vi "Main VI.vi"() -> ()   [LabVIEW 2024]
uses:
  C:/Users/user/Downloads/CarWash-master/CarWash-master/Controls/Wash Options.ctl
  C:/Users/user/Downloads/assignmentFINALHAHA/assignment/TIMEGLOBAL.vi
panel:
  out "Elapsed Time":dbl format="%#.2f"
  out "9. Vehicle Out of Position":bool
  out "8. Air Dry":bool
  out "7. Tire Shine Foam":bool
  out "6. Spot Free Rinse":bool
  out "5. Low Pressure Wax":bool
  out "4. High Pressure Wash":bool
  out "3. Pre-Soak":bool
  out "2. Bug Remover":bool
  out "1. Under Body Wash":bool
  out "Wash Entry":bool
  in  "Start":bool
  in  "Wash Options":T1
  in  "stop program":bool
  in  "Car Position Slider":u8(slide) max=3 scale=0.0..4.0
  # "Car Position Simulation"
  # "Pre-Soak\nH-P Wash\nL-P Wax\nSpot Free Rinse"
  # "Underbody Wash\nBug Remover"
  # "Tire Shine\nAir Dry"
  # "Car Wash Display"
  # "Car Wash Indicators"
  # "Entry Console"
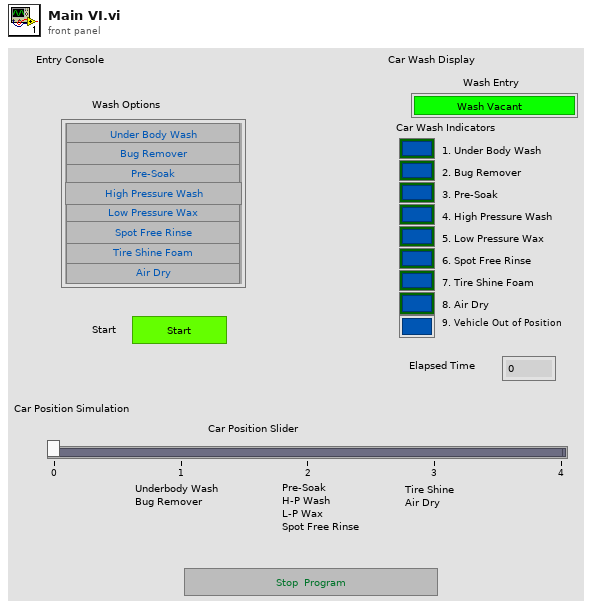
[diagram p1: front panel]
types:
  T1 = typedef "Wash Options.ctl" = cluster{"Underbody Wash":bool, "Bug Remover":bool, "Pre-Soak":bool, "High Pressure Wash":bool, "Low Pressure Wax":bool, "Spot Free Rinse":bool, "Tire Shine Foam":bool, "Air Dry":bool}
  T2 = enum16{"init", "Wait for Start", "Check Position", "under body wash", "bug remover", "pre-soak", "high pressure wash", "low pressure wax", "spot free rinse", "tire shine foam", "air dry", "Check Completion", "Log Data", "Stop Program"}
  T3 = enum8{"Enabled", "Disabled", "Disabled and Grayed Out"}
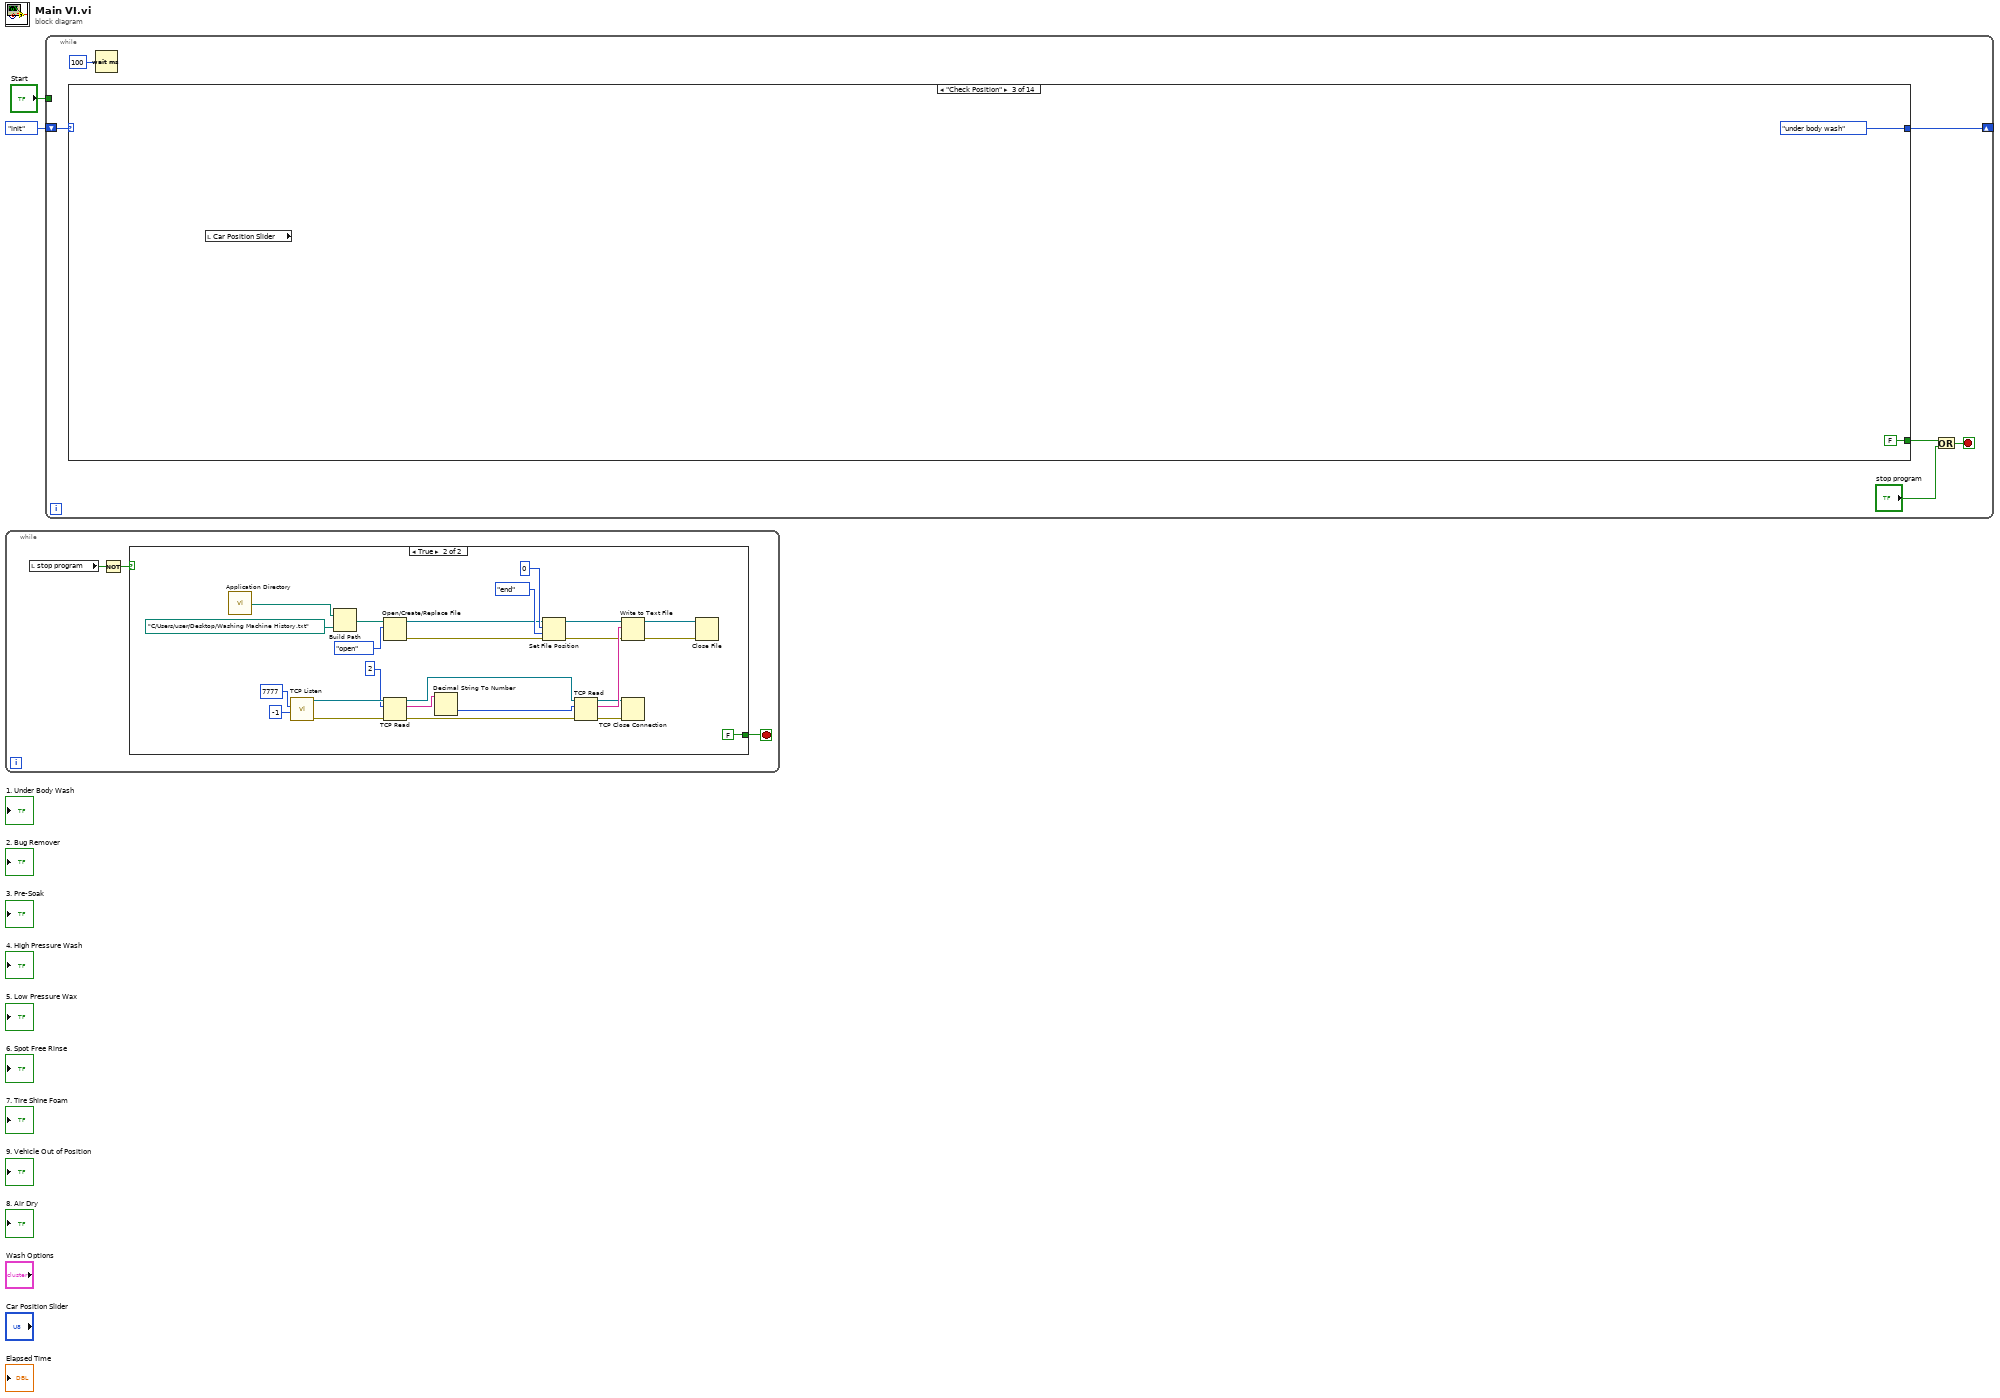
[diagram p0: block diagram]
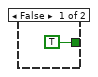
[diagram p2: hidden frame]
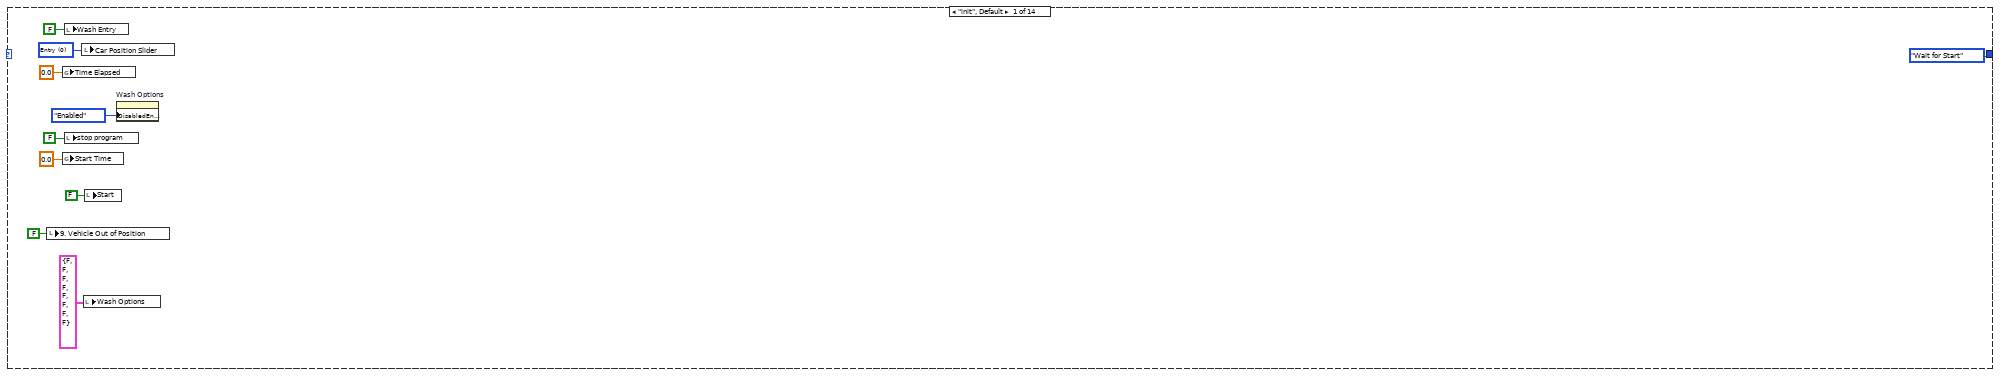
[diagram p3: hidden frame]
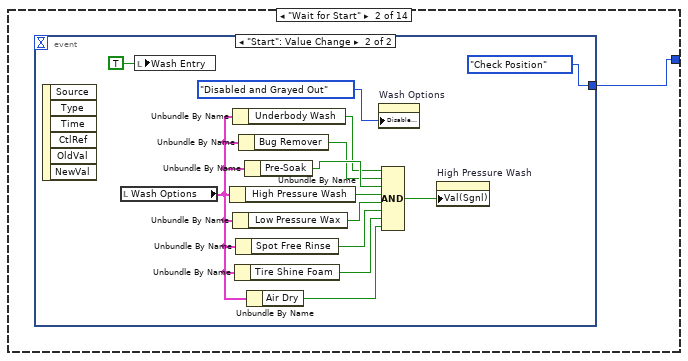
[diagram p4: hidden frame]
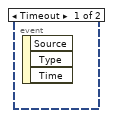
[diagram p5: hidden frame]
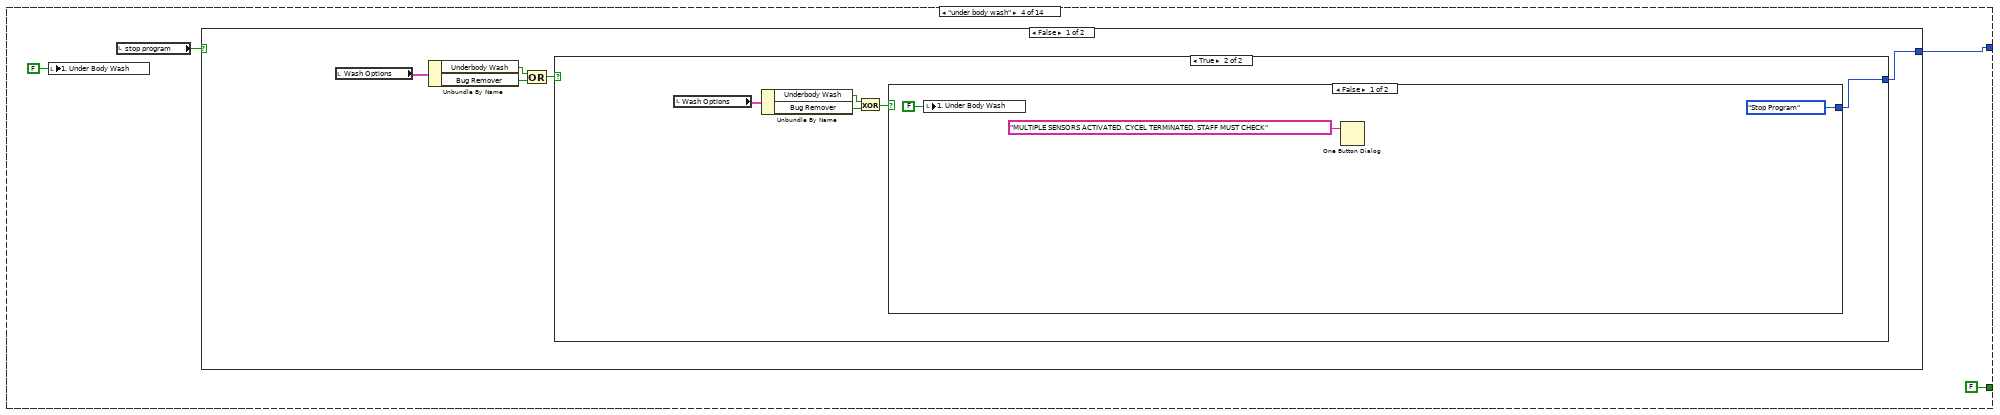
[diagram p6: hidden frame]
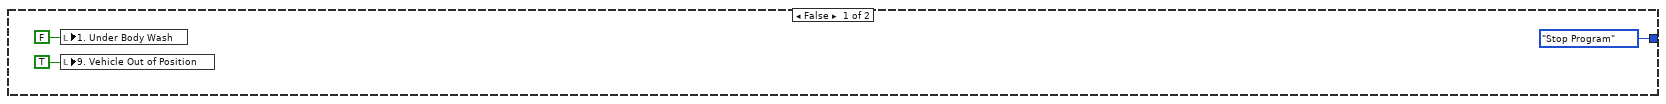
[diagram p7: hidden frame]
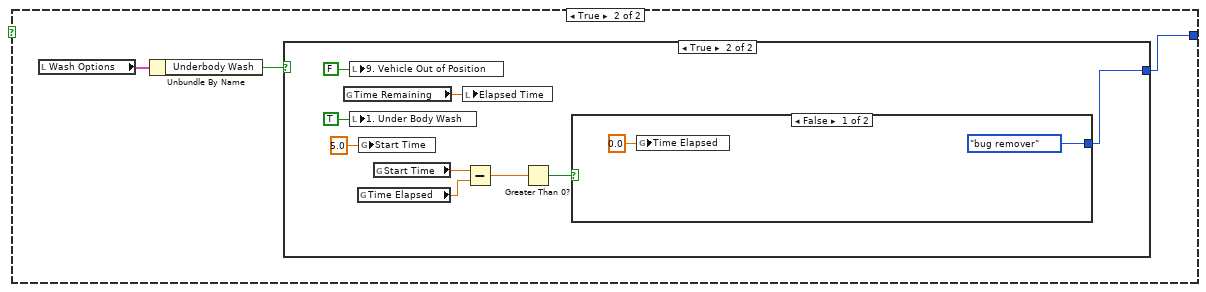
[diagram p8: hidden frame]
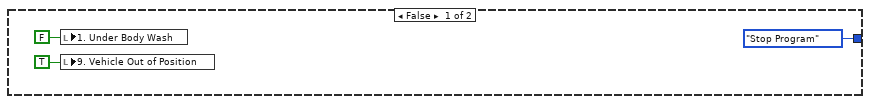
[diagram p9: hidden frame]
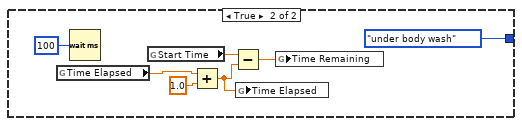
[diagram p10: hidden frame]
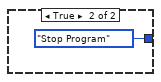
[diagram p11: hidden frame]
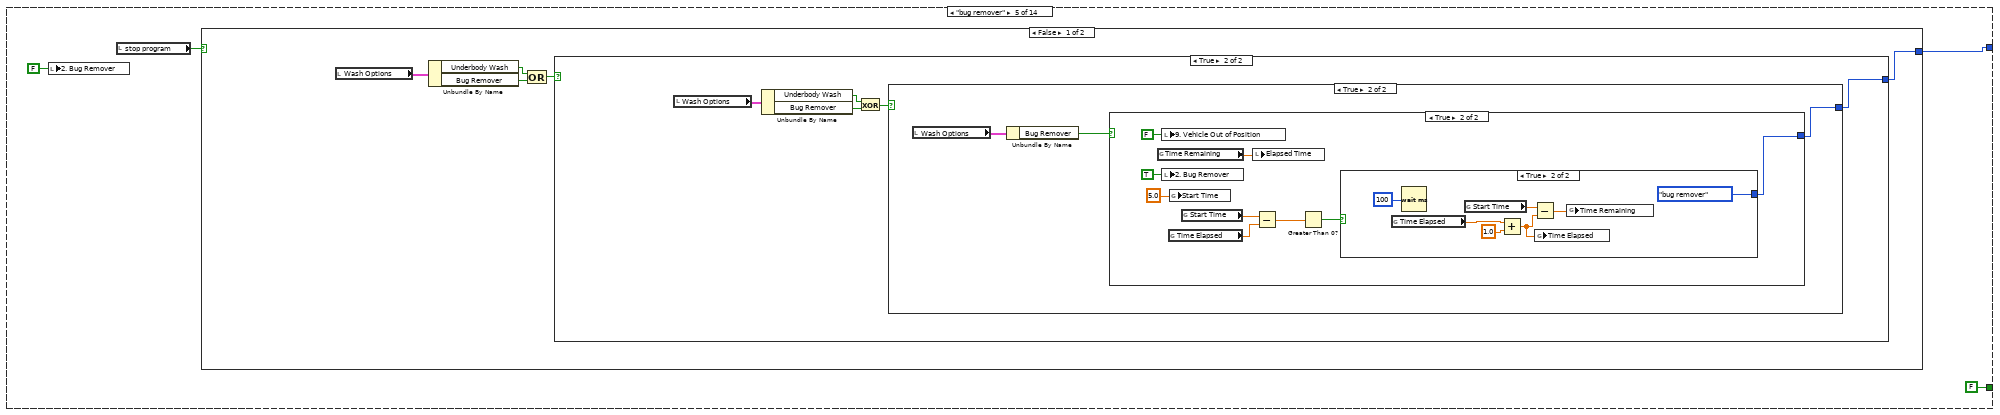
[diagram p12: hidden frame]
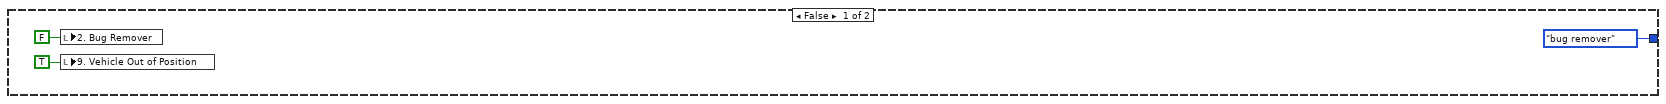
[diagram p13: hidden frame]
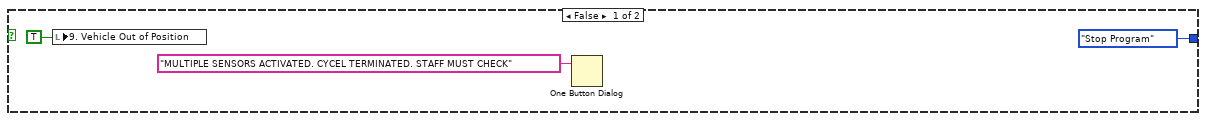
[diagram p14: hidden frame]
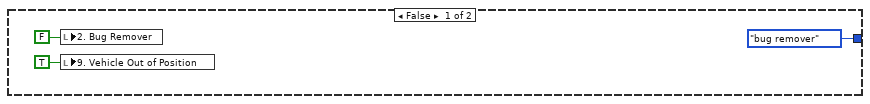
[diagram p15: hidden frame]
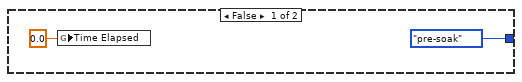
[diagram p16: hidden frame]
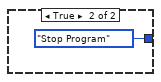
[diagram p17: hidden frame]
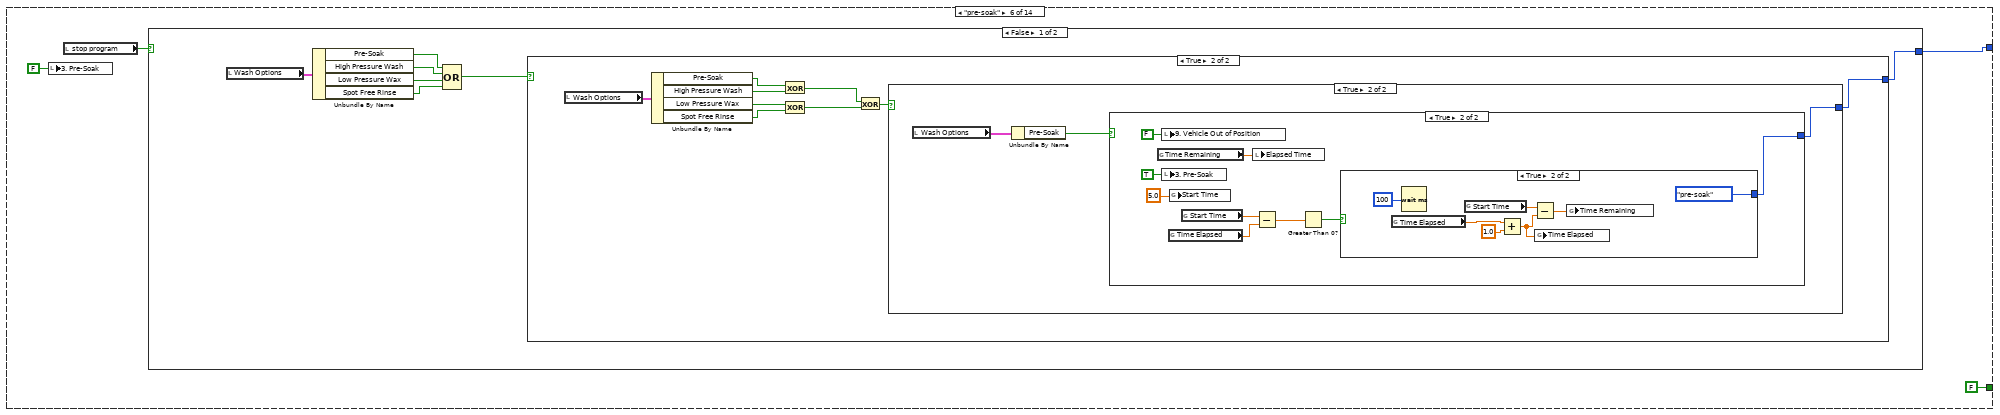
[diagram p18: hidden frame]
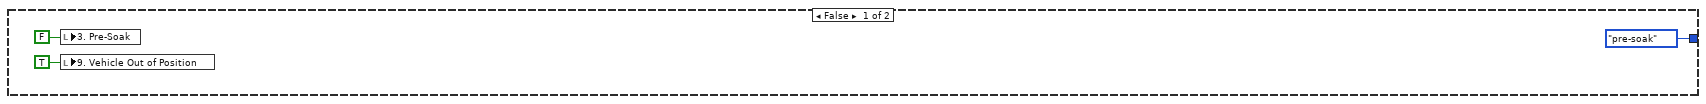
[diagram p19: hidden frame]
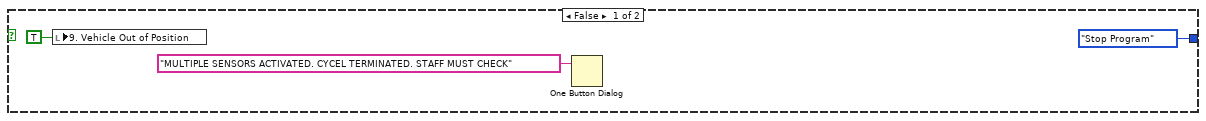
[diagram p20: hidden frame]
diagram:
  n1 = while {
    stop <- w5 stop-if-true
    n2 = local read "stop program"() -> (w3:bool)
    n3 = Not(x=w3) -> (.not. x?=w4:bool)
    n4 = case shown="True" w4 {
      tunnel: [TRUE FALSE] -> w5
      frame False {
      }
      frame True {
        n5 = call <vilib>:"Application Directory.vi"() -> ("Application Directory"=w19:path)
        n6 = call <vilib>:"TCP Listen.vi"("timeout ms (wait forever: -1)"=-1, "port"=u16 7777) -> ("error out"=w14:errorcluster, "connection ID"=w11:refnum<k5>)  [unwired: 5 in, 3 out]
        n7 = Build Path(base path=w19, name or relative path=path "C:/Users/user/Desktop/Washing Machine History.txt") -> (appended path=w31:path)
        n8 = Open/Create/Replace File(file path (use dialog)=w31, operation (0:open)=enum16{"open"}."open") -> (refnum out=w23:refnum<file>, error out=w22:errorcluster)  [unwired: 4 in, 1 out]
        n9 = TCP Read(connection ID=w11, bytes to read=2, error in (no error)=w14) -> (connection ID out=w12:refnum<k5>, data out=w17:string, error out=w15:errorcluster)  [unwired: 2 in]
        n10 = Decimal String To Number(string=w17) -> (number=w18:i32)  [unwired: 2 in, 1 out]
        n11 = Set File Position(offset (in bytes) (0)=i64 0, refnum=w23, from (0:start)=enum16{"start", "end", "current"}."end", error in=w22) -> (refnum out=w26:refnum<file>, error out=w27:errorcluster)
        n12 = TCP Read(connection ID=w12, bytes to read=w18, error in (no error)=w15) -> (connection ID out=w13:refnum<k5>, data out=w28:string, error out=w16:errorcluster)  [unwired: 2 in]
        n13 = Write to Text File(file (use dialog)=w26, text=w28, error in=w27) -> (refnum out=w29:refnum<file>, error out=w30:errorcluster)  [unwired: 1 in, 1 out]
        n14 = TCP Close Connection(connection ID=w13, error in (no error)=w16) -> ()  [unwired: 1 in, 2 out]
        n15 = Close File(refnum=w29, error in=w30) -> ()  [unwired: 2 out]
      }
    }
  }
  n16 = while {
    shift-right: [w32] -> _
    shift-left: T2."init" -> [w33]
    tunnel: "Start" -> [_]
    stop <- w35 stop-if-true
    n17 = case shown="\"Check Position\"" w33 {
      selector: w33 -> [_ _ _ _ _ _ _ _ _ _ _ _ _ w480]
      tunnel: [_ _ FALSE FALSE FALSE FALSE FALSE FALSE FALSE FALSE FALSE FALSE FALSE TRUE] -> w34
      tunnel: [T2."Wait for Start" w48 T2."under body wash" w64 w109 w154 w205 w256 w307 w358 w403 T2."Stop Program" _ w480] -> w32
      frame "init", Default {
        w45 = u8 0 items=["Entry", "Station 1", "Station 2", "Station 3", "Exit"] ("Car Position Slider")
        n18 = local write "9. Vehicle Out of Position"(FALSE ("9. Vehicle Out of Position")) -> ()
        n19 = global write "TIMEGLOBAL.vi" "Time Elapsed"(0.0 ("Time Elapsed")) -> ()
        n20 = global write "TIMEGLOBAL.vi" "Start Time"(0.0 ("Start Time")) -> ()
        n21 = local write "Wash Entry"(FALSE ("Wash Entry")) -> ()
        n22 = local write "stop program"(FALSE ("stop program")) -> ()
        n23 = local write "Car Position Slider"(w45) -> ()
        n24 = local write "Wash Options"(T1 {"Underbody Wash"=FALSE, "Bug Remover"=FALSE, "Pre-Soak"=FALSE, "High Pressure Wash"=FALSE, "Low Pressure Wax"=FALSE, "Spot Free Rinse"=FALSE, "Tire Shine Foam"=FALSE, "Air Dry"=FALSE} ("Wash Options")) -> ()
        n25 = local write "Start"(FALSE ("Start")) -> ()
        n26 = property on="Wash Options" class="Clust (strict)"("DisabledEnum"=T3."Enabled" ("Disabled")) -> ()  [unwired: 2 in, 2 out]
      }
      frame "Wait for Start" {
        n27 = event shown="[1] \"Start\": Value Change" {
          selector: _ -> [_ _]
          dyn-events: _ -> [_ _]
          timeout: _ -> [_ _]
          tunnel: [_ T2."Check Position"] -> w48
          event Timeout {
            n28 = event-data() -> ()  [unwired: 1 in, 3 out]
          }
          event "Start": Value Change {
            n29 = event-data() -> ()  [unwired: 1 in, 6 out]
            n30 = local read "Wash Options"() -> (w59:T1)
            n31 = local write "Wash Entry"(TRUE ("Wash Entry")) -> ()
            n32 = Unbundle By Name(w59) -> ("High Pressure Wash"=w53:bool)
            n33 = Unbundle By Name(w59) -> ("Underbody Wash"=w51:bool)
            n34 = Unbundle By Name(w59) -> ("Low Pressure Wax"=w55:bool)
            n35 = Unbundle By Name(w59) -> ("Tire Shine Foam"=w57:bool)
            n36 = Unbundle By Name(w59) -> ("Spot Free Rinse"=w56:bool)
            n37 = Unbundle By Name(w59) -> ("Bug Remover"=w52:bool)
            n38 = Unbundle By Name(w59) -> ("Pre-Soak"=w54:bool)
            n39 = Unbundle By Name(w59) -> ("Air Dry"=w58:bool)
            n40 = property on="Wash Options" class="Clust (strict)"("DisabledEnum"=T3."Disabled and Grayed Out" ("Disabled")) -> ()  [unwired: 2 in, 2 out]
            n41 = Compound Arithmetic op=AND(w51, w52, w54, w53, w55, w56, w57, w58) -> (w50:bool)
            n42 = property on="High Pressure Wash" class="Bool (strict)"("Val(Sgnl)"=w50) -> ()  [unwired: 2 in, 2 out]
          }
        }
      }
      frame "Check Position" {
        n43 = local read "Car Position Slider"() -> ()  [unwired: 1 out]
      }
      frame "under body wash" {
        n44 = local write "1. Under Body Wash"(FALSE ("1. Under Body Wash")) -> ()
        n45 = local read "stop program"() -> (w67:bool)
        n46 = case shown="False" w67 {
          tunnel: [w68 T2."Stop Program"] -> w64
          frame False {
            n47 = local read "Wash Options"() -> (w69:T1)
            n48 = Unbundle By Name(w69) -> ("Underbody Wash"=w71:bool, "Bug Remover"=w70:bool)
            n49 = Compound Arithmetic op=OR(w71, w70) -> (w72:bool)
            n50 = case shown="True" w72 {
              tunnel: [T2."Stop Program" w76] -> w68
              frame False {
                n51 = local write "1. Under Body Wash"(FALSE ("1. Under Body Wash")) -> ()
                n52 = local write "9. Vehicle Out of Position"(TRUE ("1. Under Body Wash")) -> ()
              }
              frame True {
                n53 = local read "Wash Options"() -> (w80:T1)
                n54 = Unbundle By Name(w80) -> ("Underbody Wash"=w79:bool, "Bug Remover"=w78:bool)
                n55 = Exclusive Or(1:w78, 2:w79) -> (0:w77:bool)
                n56 = case shown="False" w77 {
                  tunnel: [T2."Stop Program" w84] -> w76
                  frame False {
                    n57 = local write "1. Under Body Wash"(FALSE ("1. Under Body Wash")) -> ()
                    n58 = One Button Dialog(message="MULTIPLE SENSORS ACTIVATED. CYCEL TERMINATED. STAFF MUST CHECK") -> ()  [unwired: 1 in, 1 out]
                  }
                  frame True {
                    n59 = local read "Wash Options"() -> (w86:T1)
                    n60 = Unbundle By Name(w86) -> ("Underbody Wash"=w85:bool)
                    n61 = case shown="True" w85 {
                      tunnel: [T2."Stop Program" w90] -> w84
                      frame False {
                        n62 = local write "1. Under Body Wash"(FALSE ("1. Under Body Wash")) -> ()
                        n63 = local write "9. Vehicle Out of Position"(TRUE ("1. Under Body Wash")) -> ()
                      }
                      frame True {
                        n64 = global read "TIMEGLOBAL.vi" "Time Remaining"() -> (w97:dbl)
                        n65 = local write "9. Vehicle Out of Position"(FALSE ("9. Vehicle Out of Position")) -> ()
                        n66 = local write "1. Under Body Wash"(TRUE ("1. Under Body Wash")) -> ()
                        n67 = global read "TIMEGLOBAL.vi" "Time Elapsed"() -> (w95:dbl)
                        n68 = global write "TIMEGLOBAL.vi" "Start Time"(5.0 ("Start Time")) -> ()
                        n69 = global read "TIMEGLOBAL.vi" "Start Time"() -> (w94:dbl)
                        n70 = local write "Elapsed Time"(w97) -> ()
                        n71 = Subtract(x=w94, y=w95) -> (x-y=w92:dbl)
                        n72 = Greater Than 0?(x=w92) -> (x > 0?=w93:bool)
                        n73 = case shown="False" w93 {
                          tunnel: [T2."bug remover" T2."under body wash"] -> w90
                          frame False {
                            n74 = global write "TIMEGLOBAL.vi" "Time Elapsed"(0.0 ("Time Elapsed")) -> ()
                          }
                          frame True {
                            n75 = global read "TIMEGLOBAL.vi" "Time Elapsed"() -> (w104:dbl)
                            n76 = Wait (ms)(milliseconds to wait=u32 100) -> ()  [unwired: 1 out]
                            n77 = global read "TIMEGLOBAL.vi" "Start Time"() -> (w105:dbl)
                            n78 = Add(x=w104, y=1.0) -> (x+y=w103:dbl)
                            n79 = Subtract(x=w105, y=w103) -> (x-y=w102:dbl)
                            n80 = global write "TIMEGLOBAL.vi" "Time Elapsed"(w103) -> ()
                            n81 = global write "TIMEGLOBAL.vi" "Time Remaining"(w102) -> ()
                          }
                        }
                      }
                    }
                  }
                }
              }
            }
          }
          frame True {
          }
        }
      }
      frame "bug remover" {
        n82 = local write "2. Bug Remover"(FALSE ("1. Under Body Wash")) -> ()
        n83 = local read "stop program"() -> (w112:bool)
        n84 = case shown="False" w112 {
          tunnel: [w113 T2."Stop Program"] -> w109
          frame False {
            n85 = local read "Wash Options"() -> (w117:T1)
            n86 = Unbundle By Name(w117) -> ("Underbody Wash"=w115:bool, "Bug Remover"=w116:bool)
            n87 = Compound Arithmetic op=OR(w115, w116) -> (w114:bool)
            n88 = case shown="True" w114 {
              tunnel: [T2."bug remover" w121] -> w113
              frame False {
                n89 = local write "2. Bug Remover"(FALSE ("1. Under Body Wash")) -> ()
                n90 = local write "9. Vehicle Out of Position"(TRUE ("1. Under Body Wash")) -> ()
              }
              frame True {
                n91 = local read "Wash Options"() -> (w125:T1)
                n92 = Unbundle By Name(w125) -> ("Underbody Wash"=w124:bool, "Bug Remover"=w123:bool)
                n93 = Exclusive Or(1:w123, 2:w124) -> (0:w122:bool)
                n94 = case shown="True" w122 {
                  tunnel: [T2."Stop Program" w129] -> w121
                  frame False {
                    n95 = local write "9. Vehicle Out of Position"(TRUE ("1. Under Body Wash")) -> ()
                    n96 = One Button Dialog(message="MULTIPLE SENSORS ACTIVATED. CYCEL TERMINATED. STAFF MUST CHECK") -> ()  [unwired: 1 in, 1 out]
                  }
                  frame True {
                    n97 = local read "Wash Options"() -> (w131:T1)
                    n98 = Unbundle By Name(w131) -> ("Bug Remover"=w130:bool)
                    n99 = case shown="True" w130 {
                      tunnel: [T2."bug remover" w135] -> w129
                      frame False {
                        n100 = local write "2. Bug Remover"(FALSE ("1. Under Body Wash")) -> ()
                        n101 = local write "9. Vehicle Out of Position"(TRUE ("1. Under Body Wash")) -> ()
                      }
                      frame True {
                        n102 = global read "TIMEGLOBAL.vi" "Time Remaining"() -> (w142:dbl)
                        n103 = local write "9. Vehicle Out of Position"(FALSE ("9. Vehicle Out of Position")) -> ()
                        n104 = local write "2. Bug Remover"(TRUE ("1. Under Body Wash")) -> ()
                        n105 = global read "TIMEGLOBAL.vi" "Time Elapsed"() -> (w140:dbl)
                        n106 = global write "TIMEGLOBAL.vi" "Start Time"(5.0 ("Start Time")) -> ()
                        n107 = global read "TIMEGLOBAL.vi" "Start Time"() -> (w139:dbl)
                        n108 = local write "Elapsed Time"(w142) -> ()
                        n109 = Subtract(x=w139, y=w140) -> (x-y=w137:dbl)
                        n110 = Greater Than 0?(x=w137) -> (x > 0?=w138:bool)
                        n111 = case shown="True" w138 {
                          tunnel: [T2."pre-soak" T2."bug remover"] -> w135
                          frame False {
                            n112 = global write "TIMEGLOBAL.vi" "Time Elapsed"(0.0 ("Time Elapsed")) -> ()
                          }
                          frame True {
                            n113 = global read "TIMEGLOBAL.vi" "Time Elapsed"() -> (w149:dbl)
                            n114 = Wait (ms)(milliseconds to wait=u32 100) -> ()  [unwired: 1 out]
                            n115 = global read "TIMEGLOBAL.vi" "Start Time"() -> (w150:dbl)
                            n116 = Add(x=w149, y=1.0) -> (x+y=w148:dbl)
                            n117 = Subtract(x=w150, y=w148) -> (x-y=w147:dbl)
                            n118 = global write "TIMEGLOBAL.vi" "Time Elapsed"(w148) -> ()
                            n119 = global write "TIMEGLOBAL.vi" "Time Remaining"(w147) -> ()
                          }
                        }
                      }
                    }
                  }
                }
              }
            }
          }
          frame True {
          }
        }
      }
      frame "pre-soak" {
        n120 = local write "3. Pre-Soak"(FALSE ("1. Under Body Wash")) -> ()
        n121 = local read "stop program"() -> (w157:bool)
        n122 = case shown="False" w157 {
          tunnel: [w158 T2."Stop Program"] -> w154
          frame False {
            n123 = local read "Wash Options"() -> (w163:T1)
            n124 = Unbundle By Name(w163) -> ("Pre-Soak"=w162:bool, "High Pressure Wash"=w161:bool, "Low Pressure Wax"=w160:bool, "Spot Free Rinse"=w159:bool)
            n125 = Compound Arithmetic op=OR(w162, w161, w160, w159) -> (w164:bool)
            n126 = case shown="True" w164 {
              tunnel: [T2."pre-soak" w168] -> w158
              frame False {
                n127 = local write "3. Pre-Soak"(FALSE ("1. Under Body Wash")) -> ()
                n128 = local write "9. Vehicle Out of Position"(TRUE ("1. Under Body Wash")) -> ()
              }
              frame True {
                n129 = local read "Wash Options"() -> (w173:T1)
                n130 = Unbundle By Name(w173) -> ("Pre-Soak"=w172:bool, "High Pressure Wash"=w171:bool, "Low Pressure Wax"=w170:bool, "Spot Free Rinse"=w169:bool)
                n131 = Exclusive Or(1:w171, 2:w172) -> (0:w175:bool)
                n132 = Exclusive Or(1:w169, 2:w170) -> (0:w176:bool)
                n133 = Exclusive Or(1:w176, 2:w175) -> (0:w174:bool)
                n134 = case shown="True" w174 {
                  tunnel: [T2."Stop Program" w180] -> w168
                  frame False {
                    n135 = local write "9. Vehicle Out of Position"(TRUE ("1. Under Body Wash")) -> ()
                    n136 = One Button Dialog(message="MULTIPLE SENSORS ACTIVATED. CYCEL TERMINATED. STAFF MUST CHECK") -> ()  [unwired: 1 in, 1 out]
                  }
                  frame True {
                    n137 = local read "Wash Options"() -> (w182:T1)
                    n138 = Unbundle By Name(w182) -> ("Pre-Soak"=w181:bool)
                    n139 = case shown="True" w181 {
                      tunnel: [T2."pre-soak" w186] -> w180
                      frame False {
                        n140 = local write "3. Pre-Soak"(FALSE ("1. Under Body Wash")) -> ()
                        n141 = local write "9. Vehicle Out of Position"(TRUE ("1. Under Body Wash")) -> ()
                      }
                      frame True {
                        n142 = global read "TIMEGLOBAL.vi" "Time Remaining"() -> (w193:dbl)
                        n143 = local write "9. Vehicle Out of Position"(FALSE ("9. Vehicle Out of Position")) -> ()
                        n144 = local write "3. Pre-Soak"(TRUE ("1. Under Body Wash")) -> ()
                        n145 = global read "TIMEGLOBAL.vi" "Time Elapsed"() -> (w191:dbl)
                        n146 = global write "TIMEGLOBAL.vi" "Start Time"(5.0 ("Start Time")) -> ()
                        n147 = global read "TIMEGLOBAL.vi" "Start Time"() -> (w190:dbl)
                        n148 = local write "Elapsed Time"(w193) -> ()
                        n149 = Subtract(x=w190, y=w191) -> (x-y=w188:dbl)
                        n150 = Greater Than 0?(x=w188) -> (x > 0?=w189:bool)
                        n151 = case shown="True" w189 {
                          tunnel: [T2."high pressure wash" T2."pre-soak"] -> w186
                          frame False {
                            n152 = global write "TIMEGLOBAL.vi" "Time Elapsed"(0.0 ("Time Elapsed")) -> ()
                          }
                          frame True {
                            n153 = global read "TIMEGLOBAL.vi" "Time Elapsed"() -> (w200:dbl)
                            n154 = Wait (ms)(milliseconds to wait=u32 100) -> ()  [unwired: 1 out]
                            n155 = global read "TIMEGLOBAL.vi" "Start Time"() -> (w201:dbl)
                            n156 = Add(x=w200, y=1.0) -> (x+y=w199:dbl)
                            n157 = Subtract(x=w201, y=w199) -> (x-y=w198:dbl)
                            n158 = global write "TIMEGLOBAL.vi" "Time Elapsed"(w199) -> ()
                            n159 = global write "TIMEGLOBAL.vi" "Time Remaining"(w198) -> ()
                          }
                        }
                      }
                    }
                  }
                }
              }
            }
          }
          frame True {
          }
        }
      }
      frame "high pressure wash" {
        n160 = local write "4. High Pressure Wash"(FALSE ("1. Under Body Wash")) -> ()
        n161 = local read "stop program"() -> (w208:bool)
        n162 = case shown="False" w208 {
          tunnel: [w209 T2."Stop Program"] -> w205
          frame False {
            n163 = local read "Wash Options"() -> (w214:T1)
            n164 = Unbundle By Name(w214) -> ("Pre-Soak"=w213:bool, "High Pressure Wash"=w212:bool, "Low Pressure Wax"=w211:bool, "Spot Free Rinse"=w210:bool)
            n165 = Compound Arithmetic op=OR(w213, w212, w211, w210) -> (w215:bool)
            n166 = case shown="True" w215 {
              tunnel: [T2."high pressure wash" w219] -> w209
              frame False {
                n167 = local write "4. High Pressure Wash"(FALSE ("1. Under Body Wash")) -> ()
                n168 = local write "9. Vehicle Out of Position"(TRUE ("1. Under Body Wash")) -> ()
              }
              frame True {
                n169 = local read "Wash Options"() -> (w224:T1)
                n170 = Unbundle By Name(w224) -> ("Pre-Soak"=w223:bool, "High Pressure Wash"=w222:bool, "Low Pressure Wax"=w221:bool, "Spot Free Rinse"=w220:bool)
                n171 = Exclusive Or(1:w222, 2:w223) -> (0:w226:bool)
                n172 = Exclusive Or(1:w220, 2:w221) -> (0:w227:bool)
                n173 = Exclusive Or(1:w227, 2:w226) -> (0:w225:bool)
                n174 = case shown="True" w225 {
                  tunnel: [T2."Stop Program" w231] -> w219
                  frame False {
                    n175 = local write "9. Vehicle Out of Position"(TRUE ("1. Under Body Wash")) -> ()
                    n176 = One Button Dialog(message="MULTIPLE SENSORS ACTIVATED. CYCEL TERMINATED. STAFF MUST CHECK") -> ()  [unwired: 1 in, 1 out]
                  }
                  frame True {
                    n177 = local read "Wash Options"() -> (w233:T1)
                    n178 = Unbundle By Name(w233) -> ("High Pressure Wash"=w232:bool)
                    n179 = case shown="True" w232 {
                      tunnel: [T2."high pressure wash" w237] -> w231
                      frame False {
                        n180 = local write "4. High Pressure Wash"(FALSE ("1. Under Body Wash")) -> ()
                        n181 = local write "9. Vehicle Out of Position"(TRUE ("1. Under Body Wash")) -> ()
                      }
                      frame True {
                        n182 = global read "TIMEGLOBAL.vi" "Time Remaining"() -> (w244:dbl)
                        n183 = local write "9. Vehicle Out of Position"(FALSE ("9. Vehicle Out of Position")) -> ()
                        n184 = local write "4. High Pressure Wash"(TRUE ("1. Under Body Wash")) -> ()
                        n185 = global read "TIMEGLOBAL.vi" "Time Elapsed"() -> (w242:dbl)
                        n186 = global write "TIMEGLOBAL.vi" "Start Time"(5.0 ("Start Time")) -> ()
                        n187 = global read "TIMEGLOBAL.vi" "Start Time"() -> (w241:dbl)
                        n188 = local write "Elapsed Time"(w244) -> ()
                        n189 = Subtract(x=w241, y=w242) -> (x-y=w239:dbl)
                        n190 = Greater Than 0?(x=w239) -> (x > 0?=w240:bool)
                        n191 = case shown="True" w240 {
                          tunnel: [T2."low pressure wax" T2."high pressure wash"] -> w237
                          frame False {
                            n192 = global write "TIMEGLOBAL.vi" "Time Elapsed"(0.0 ("Time Elapsed")) -> ()
                          }
                          frame True {
                            n193 = global read "TIMEGLOBAL.vi" "Time Elapsed"() -> (w251:dbl)
                            n194 = Wait (ms)(milliseconds to wait=u32 100) -> ()  [unwired: 1 out]
                            n195 = global read "TIMEGLOBAL.vi" "Start Time"() -> (w252:dbl)
                            n196 = Add(x=w251, y=1.0) -> (x+y=w250:dbl)
                            n197 = Subtract(x=w252, y=w250) -> (x-y=w249:dbl)
                            n198 = global write "TIMEGLOBAL.vi" "Time Elapsed"(w250) -> ()
                            n199 = global write "TIMEGLOBAL.vi" "Time Remaining"(w249) -> ()
                          }
                        }
                      }
                    }
                  }
                }
              }
            }
          }
          frame True {
          }
        }
      }
      frame "low pressure wax" {
        n200 = local write "5. Low Pressure Wax"(FALSE ("1. Under Body Wash")) -> ()
        n201 = local read "stop program"() -> (w259:bool)
        n202 = case shown="False" w259 {
          tunnel: [w260 T2."Stop Program"] -> w256
          frame False {
            n203 = local read "Wash Options"() -> (w265:T1)
            n204 = Unbundle By Name(w265) -> ("Pre-Soak"=w264:bool, "High Pressure Wash"=w263:bool, "Low Pressure Wax"=w262:bool, "Spot Free Rinse"=w261:bool)
            n205 = Compound Arithmetic op=OR(w264, w263, w262, w261) -> (w266:bool)
            n206 = case shown="True" w266 {
              tunnel: [T2."low pressure wax" w270] -> w260
              frame False {
                n207 = local write "5. Low Pressure Wax"(FALSE ("1. Under Body Wash")) -> ()
                n208 = local write "9. Vehicle Out of Position"(TRUE ("1. Under Body Wash")) -> ()
              }
              frame True {
                n209 = local read "Wash Options"() -> (w275:T1)
                n210 = Unbundle By Name(w275) -> ("Pre-Soak"=w274:bool, "High Pressure Wash"=w273:bool, "Low Pressure Wax"=w272:bool, "Spot Free Rinse"=w271:bool)
                n211 = Exclusive Or(1:w273, 2:w274) -> (0:w277:bool)
                n212 = Exclusive Or(1:w271, 2:w272) -> (0:w278:bool)
                n213 = Exclusive Or(1:w278, 2:w277) -> (0:w276:bool)
                n214 = case shown="True" w276 {
                  tunnel: [T2."Stop Program" w282] -> w270
                  frame False {
                    n215 = local write "9. Vehicle Out of Position"(TRUE ("1. Under Body Wash")) -> ()
                    n216 = One Button Dialog(message="MULTIPLE SENSORS ACTIVATED. CYCEL TERMINATED. STAFF MUST CHECK") -> ()  [unwired: 1 in, 1 out]
                  }
                  frame True {
                    n217 = local read "Wash Options"() -> (w284:T1)
                    n218 = Unbundle By Name(w284) -> ("Low Pressure Wax"=w283:bool)
                    n219 = case shown="True" w283 {
                      tunnel: [T2."low pressure wax" w288] -> w282
                      frame False {
                        n220 = local write "5. Low Pressure Wax"(FALSE ("1. Under Body Wash")) -> ()
                        n221 = local write "9. Vehicle Out of Position"(TRUE ("1. Under Body Wash")) -> ()
                      }
                      frame True {
                        n222 = global read "TIMEGLOBAL.vi" "Time Remaining"() -> (w295:dbl)
                        n223 = local write "9. Vehicle Out of Position"(FALSE ("9. Vehicle Out of Position")) -> ()
                        n224 = local write "5. Low Pressure Wax"(TRUE ("1. Under Body Wash")) -> ()
                        n225 = global read "TIMEGLOBAL.vi" "Time Elapsed"() -> (w293:dbl)
                        n226 = global write "TIMEGLOBAL.vi" "Start Time"(5.0 ("Start Time")) -> ()
                        n227 = global read "TIMEGLOBAL.vi" "Start Time"() -> (w292:dbl)
                        n228 = local write "Elapsed Time"(w295) -> ()
                        n229 = Subtract(x=w292, y=w293) -> (x-y=w290:dbl)
                        n230 = Greater Than 0?(x=w290) -> (x > 0?=w291:bool)
                        n231 = case shown="True" w291 {
                          tunnel: [T2."high pressure wash" T2."low pressure wax"] -> w288
                          frame False {
                            n232 = global write "TIMEGLOBAL.vi" "Time Elapsed"(0.0 ("Time Elapsed")) -> ()
                          }
                          frame True {
                            n233 = global read "TIMEGLOBAL.vi" "Time Elapsed"() -> (w302:dbl)
                            n234 = Wait (ms)(milliseconds to wait=u32 100) -> ()  [unwired: 1 out]
                            n235 = global read "TIMEGLOBAL.vi" "Start Time"() -> (w303:dbl)
                            n236 = Add(x=w302, y=1.0) -> (x+y=w301:dbl)
                            n237 = Subtract(x=w303, y=w301) -> (x-y=w300:dbl)
                            n238 = global write "TIMEGLOBAL.vi" "Time Elapsed"(w301) -> ()
                            n239 = global write "TIMEGLOBAL.vi" "Time Remaining"(w300) -> ()
                          }
                        }
                      }
                    }
                  }
                }
              }
            }
          }
          frame True {
          }
        }
      }
      frame "spot free rinse" {
        n240 = local write "6. Spot Free Rinse"(FALSE ("1. Under Body Wash")) -> ()
        n241 = local read "stop program"() -> (w310:bool)
        n242 = case shown="False" w310 {
          tunnel: [w311 T2."Stop Program"] -> w307
          frame False {
            n243 = local read "Wash Options"() -> (w316:T1)
            n244 = Unbundle By Name(w316) -> ("Pre-Soak"=w315:bool, "High Pressure Wash"=w314:bool, "Low Pressure Wax"=w313:bool, "Spot Free Rinse"=w312:bool)
            n245 = Compound Arithmetic op=OR(w315, w314, w313, w312) -> (w317:bool)
            n246 = case shown="True" w317 {
              tunnel: [T2."spot free rinse" w321] -> w311
              frame False {
                n247 = local write "6. Spot Free Rinse"(FALSE ("1. Under Body Wash")) -> ()
                n248 = local write "9. Vehicle Out of Position"(TRUE ("1. Under Body Wash")) -> ()
              }
              frame True {
                n249 = local read "Wash Options"() -> (w326:T1)
                n250 = Unbundle By Name(w326) -> ("Pre-Soak"=w325:bool, "High Pressure Wash"=w324:bool, "Low Pressure Wax"=w323:bool, "Spot Free Rinse"=w322:bool)
                n251 = Exclusive Or(1:w324, 2:w325) -> (0:w328:bool)
                n252 = Exclusive Or(1:w322, 2:w323) -> (0:w329:bool)
                n253 = Exclusive Or(1:w329, 2:w328) -> (0:w327:bool)
                n254 = case shown="True" w327 {
                  tunnel: [T2."Stop Program" w333] -> w321
                  frame False {
                    n255 = local write "9. Vehicle Out of Position"(TRUE ("1. Under Body Wash")) -> ()
                    n256 = One Button Dialog(message="MULTIPLE SENSORS ACTIVATED. CYCEL TERMINATED. STAFF MUST CHECK") -> ()  [unwired: 1 in, 1 out]
                  }
                  frame True {
                    n257 = local read "Wash Options"() -> (w335:T1)
                    n258 = Unbundle By Name(w335) -> ("Spot Free Rinse"=w334:bool)
                    n259 = case shown="True" w334 {
                      tunnel: [T2."spot free rinse" w339] -> w333
                      frame False {
                        n260 = local write "6. Spot Free Rinse"(FALSE ("1. Under Body Wash")) -> ()
                        n261 = local write "9. Vehicle Out of Position"(TRUE ("1. Under Body Wash")) -> ()
                      }
                      frame True {
                        n262 = global read "TIMEGLOBAL.vi" "Time Remaining"() -> (w346:dbl)
                        n263 = local write "9. Vehicle Out of Position"(FALSE ("9. Vehicle Out of Position")) -> ()
                        n264 = local write "6. Spot Free Rinse"(TRUE ("1. Under Body Wash")) -> ()
                        n265 = global read "TIMEGLOBAL.vi" "Time Elapsed"() -> (w344:dbl)
                        n266 = global write "TIMEGLOBAL.vi" "Start Time"(5.0 ("Start Time")) -> ()
                        n267 = global read "TIMEGLOBAL.vi" "Start Time"() -> (w343:dbl)
                        n268 = local write "Elapsed Time"(w346) -> ()
                        n269 = Subtract(x=w343, y=w344) -> (x-y=w341:dbl)
                        n270 = Greater Than 0?(x=w341) -> (x > 0?=w342:bool)
                        n271 = case shown="True" w342 {
                          tunnel: [T2."tire shine foam" T2."spot free rinse"] -> w339
                          frame False {
                            n272 = global write "TIMEGLOBAL.vi" "Time Elapsed"(0.0 ("Time Elapsed")) -> ()
                          }
                          frame True {
                            n273 = global read "TIMEGLOBAL.vi" "Time Elapsed"() -> (w353:dbl)
                            n274 = Wait (ms)(milliseconds to wait=u32 100) -> ()  [unwired: 1 out]
                            n275 = global read "TIMEGLOBAL.vi" "Start Time"() -> (w354:dbl)
                            n276 = Add(x=w353, y=1.0) -> (x+y=w352:dbl)
                            n277 = Subtract(x=w354, y=w352) -> (x-y=w351:dbl)
                            n278 = global write "TIMEGLOBAL.vi" "Time Elapsed"(w352) -> ()
                            n279 = global write "TIMEGLOBAL.vi" "Time Remaining"(w351) -> ()
                          }
                        }
                      }
                    }
                  }
                }
              }
            }
          }
          frame True {
          }
        }
      }
      frame "tire shine foam" {
        n280 = local write "7. Tire Shine Foam"(FALSE ("1. Under Body Wash")) -> ()
        n281 = local read "stop program"() -> (w361:bool)
        n282 = case shown="False" w361 {
          tunnel: [w362 T2."Stop Program"] -> w358
          frame False {
            n283 = local read "Wash Options"() -> (w365:T1)
            n284 = Unbundle By Name(w365) -> ("Tire Shine Foam"=w364:bool, "Air Dry"=w363:bool)
            n285 = Compound Arithmetic op=OR(w364, w363) -> (w366:bool)
            n286 = case shown="True" w366 {
              tunnel: [T2."tire shine foam" w370] -> w362
              frame False {
                n287 = local write "7. Tire Shine Foam"(FALSE ("1. Under Body Wash")) -> ()
                n288 = local write "9. Vehicle Out of Position"(TRUE ("1. Under Body Wash")) -> ()
              }
              frame True {
                n289 = local read "Wash Options"() -> (w374:T1)
                n290 = Unbundle By Name(w374) -> ("Tire Shine Foam"=w373:bool, "Air Dry"=w372:bool)
                n291 = Exclusive Or(1:w372, 2:w373) -> (0:w371:bool)
                n292 = case shown="True" w371 {
                  tunnel: [T2."Stop Program" w378] -> w370
                  frame False {
                    n293 = local write "9. Vehicle Out of Position"(TRUE ("1. Under Body Wash")) -> ()
                    n294 = One Button Dialog(message="MULTIPLE SENSORS ACTIVATED. CYCEL TERMINATED. STAFF MUST CHECK") -> ()  [unwired: 1 in, 1 out]
                  }
                  frame True {
                    n295 = local read "Wash Options"() -> (w380:T1)
                    n296 = Unbundle By Name(w380) -> ("Tire Shine Foam"=w379:bool)
                    n297 = case shown="True" w379 {
                      tunnel: [T2."tire shine foam" w384] -> w378
                      frame False {
                        n298 = local write "7. Tire Shine Foam"(FALSE ("1. Under Body Wash")) -> ()
                        n299 = local write "9. Vehicle Out of Position"(TRUE ("1. Under Body Wash")) -> ()
                      }
                      frame True {
                        n300 = global read "TIMEGLOBAL.vi" "Time Remaining"() -> (w391:dbl)
                        n301 = local write "9. Vehicle Out of Position"(FALSE ("9. Vehicle Out of Position")) -> ()
                        n302 = local write "7. Tire Shine Foam"(TRUE ("1. Under Body Wash")) -> ()
                        n303 = global read "TIMEGLOBAL.vi" "Time Elapsed"() -> (w389:dbl)
                        n304 = global write "TIMEGLOBAL.vi" "Start Time"(5.0 ("Start Time")) -> ()
                        n305 = global read "TIMEGLOBAL.vi" "Start Time"() -> (w388:dbl)
                        n306 = local write "Elapsed Time"(w391) -> ()
                        n307 = Subtract(x=w388, y=w389) -> (x-y=w386:dbl)
                        n308 = Greater Than 0?(x=w386) -> (x > 0?=w387:bool)
                        n309 = case shown="True" w387 {
                          tunnel: [T2."air dry" T2."tire shine foam"] -> w384
                          frame False {
                            n310 = global write "TIMEGLOBAL.vi" "Time Elapsed"(0.0 ("Time Elapsed")) -> ()
                          }
                          frame True {
                            n311 = global read "TIMEGLOBAL.vi" "Time Elapsed"() -> (w398:dbl)
                            n312 = Wait (ms)(milliseconds to wait=u32 100) -> ()  [unwired: 1 out]
                            n313 = global read "TIMEGLOBAL.vi" "Start Time"() -> (w399:dbl)
                            n314 = Add(x=w398, y=1.0) -> (x+y=w397:dbl)
                            n315 = Subtract(x=w399, y=w397) -> (x-y=w396:dbl)
                            n316 = global write "TIMEGLOBAL.vi" "Time Elapsed"(w397) -> ()
                            n317 = global write "TIMEGLOBAL.vi" "Time Remaining"(w396) -> ()
                          }
                        }
                      }
                    }
                  }
                }
              }
            }
          }
          frame True {
          }
        }
      }
      frame "air dry" {
        n318 = local write "8. Air Dry"(FALSE ("1. Under Body Wash")) -> ()
        n319 = local read "stop program"() -> (w406:bool)
        n320 = case shown="False" w406 {
          tunnel: [w407 T2."Stop Program"] -> w403
          frame False {
            n321 = local read "Wash Options"() -> (w410:T1)
            n322 = Unbundle By Name(w410) -> ("Tire Shine Foam"=w409:bool, "Air Dry"=w408:bool)
            n323 = Compound Arithmetic op=OR(w409, w408) -> (w411:bool)
            n324 = case shown="True" w411 {
              tunnel: [T2."air dry" w415] -> w407
              frame False {
                n325 = local write "8. Air Dry"(FALSE ("1. Under Body Wash")) -> ()
                n326 = local write "9. Vehicle Out of Position"(TRUE ("1. Under Body Wash")) -> ()
              }
              frame True {
                n327 = local read "Wash Options"() -> (w419:T1)
                n328 = Unbundle By Name(w419) -> ("Tire Shine Foam"=w418:bool, "Air Dry"=w417:bool)
                n329 = Exclusive Or(1:w417, 2:w418) -> (0:w416:bool)
                n330 = case shown="True" w416 {
                  tunnel: [T2."Stop Program" w423] -> w415
                  frame False {
                    n331 = local write "9. Vehicle Out of Position"(TRUE ("1. Under Body Wash")) -> ()
                    n332 = One Button Dialog(message="MULTIPLE SENSORS ACTIVATED. CYCEL TERMINATED. STAFF MUST CHECK") -> ()  [unwired: 1 in, 1 out]
                  }
                  frame True {
                    n333 = local read "Wash Options"() -> (w425:T1)
                    n334 = Unbundle By Name(w425) -> ("Air Dry"=w424:bool)
                    n335 = case shown="True" w424 {
                      tunnel: [T2."air dry" w429] -> w423
                      frame False {
                        n336 = local write "8. Air Dry"(FALSE ("1. Under Body Wash")) -> ()
                        n337 = local write "9. Vehicle Out of Position"(TRUE ("1. Under Body Wash")) -> ()
                      }
                      frame True {
                        n338 = global read "TIMEGLOBAL.vi" "Time Remaining"() -> (w436:dbl)
                        n339 = local write "9. Vehicle Out of Position"(FALSE ("9. Vehicle Out of Position")) -> ()
                        n340 = local write "8. Air Dry"(TRUE ("1. Under Body Wash")) -> ()
                        n341 = global read "TIMEGLOBAL.vi" "Time Elapsed"() -> (w434:dbl)
                        n342 = global write "TIMEGLOBAL.vi" "Start Time"(5.0 ("Start Time")) -> ()
                        n343 = global read "TIMEGLOBAL.vi" "Start Time"() -> (w433:dbl)
                        n344 = local write "Elapsed Time"(w436) -> ()
                        n345 = Subtract(x=w433, y=w434) -> (x-y=w431:dbl)
                        n346 = Greater Than 0?(x=w431) -> (x > 0?=w432:bool)
                        n347 = case shown="True" w432 {
                          tunnel: [T2."Check Completion" T2."air dry"] -> w429
                          frame False {
                            n348 = global write "TIMEGLOBAL.vi" "Time Elapsed"(0.0 ("Time Elapsed")) -> ()
                          }
                          frame True {
                            n349 = global read "TIMEGLOBAL.vi" "Time Elapsed"() -> (w443:dbl)
                            n350 = Wait (ms)(milliseconds to wait=u32 100) -> ()  [unwired: 1 out]
                            n351 = global read "TIMEGLOBAL.vi" "Start Time"() -> (w444:dbl)
                            n352 = Add(x=w443, y=1.0) -> (x+y=w442:dbl)
                            n353 = Subtract(x=w444, y=w442) -> (x-y=w441:dbl)
                            n354 = global write "TIMEGLOBAL.vi" "Time Elapsed"(w442) -> ()
                            n355 = global write "TIMEGLOBAL.vi" "Time Remaining"(w441) -> ()
                          }
                        }
                      }
                    }
                  }
                }
              }
            }
          }
          frame True {
          }
        }
      }
      frame "Check Completion" {
        w459 = u8 0 items=["Entry", "Station 1", "Station 2", "Station 3", "Exit"] ("Car Position Slider")
        n356 = local write "9. Vehicle Out of Position"(TRUE ("9. Vehicle Out of Position")) -> ()
        n357 = local write "8. Air Dry"(FALSE ("9. Vehicle Out of Position")) -> ()
        n358 = local write "7. Tire Shine Foam"(FALSE ("9. Vehicle Out of Position")) -> ()
        n359 = local write "6. Spot Free Rinse"(FALSE ("9. Vehicle Out of Position")) -> ()
        n360 = local write "5. Low Pressure Wax"(FALSE ("9. Vehicle Out of Position")) -> ()
        n361 = local write "4. High Pressure Wash"(FALSE ("9. Vehicle Out of Position")) -> ()
        n362 = local write "3. Pre-Soak"(FALSE ("9. Vehicle Out of Position")) -> ()
        n363 = local write "2. Bug Remover"(FALSE ("9. Vehicle Out of Position")) -> ()
        n364 = local write "1. Under Body Wash"(FALSE ("9. Vehicle Out of Position")) -> ()
        n365 = local write "Car Position Slider"(w459) -> ()
        n366 = property on="Wash Options" class="Clust (strict)"("DisabledEnum"=T3."Enabled" ("Disabled")) -> ()  [unwired: 2 in, 2 out]
        "Wash Entry" <- FALSE ("Wash Entry")
      }
      frame "Log Data" {
        n367 = Get Date/Time String() -> (date string=w469:string, time string=w464:string)  [unwired: 3 in]
        n368 = Concatenate Strings(w469, "\t" ("string"), w464, "\t" ("string"), "\r\n") -> (w468:string)
        n369 = String Length(string=w468) -> (length=w471:i32)
        n370 = Number To Decimal String(number=w471, width (-)=i16 2) -> (decimal integer string=w472:string)
        n371 = TCP Open Connection(remote port or service name=u16 7777, timeout ms (60000)=60000) -> (connection ID=w478:refnum<k5>, error out=w473:errorcluster)  [unwired: 3 in]
        n372 = TCP Write(connection ID=w478, data in=w472, error in (no error)=w473) -> (connection ID out=w477:refnum<k5>, error out=w474:errorcluster)  [unwired: 1 in, 1 out]
        n373 = TCP Write(connection ID=w477, data in=w468, error in (no error)=w474) -> (connection ID out=w476:refnum<k5>, error out=w475:errorcluster)  [unwired: 1 in, 1 out]
        n374 = TCP Close Connection(connection ID=w476, error in (no error)=w475) -> ()  [unwired: 1 in, 2 out]
      }
      frame "Stop Program" {
      }
    }
    n375 = Wait (ms)(milliseconds to wait=u32 100) -> ()  [unwired: 1 out]
    n376 = Or(x=w34, y="stop program") -> (x .or. y?=w35:bool)
  }
